vi "Fixated.vi"(10 "Input":variant, 11 "Data":T1) -> (2 "Fixated":bool, 3 "Adjustment":dbl[](array[numeric]))   [LabVIEW 2010]
uses:
  Core SubVIs/Controls/TYPE - Analog Data.ctl
  <vilib>/imath/engines/lvmath2/RunTimeEngine/ErrorHandling/NIMS_Finalize Error.vi
  <vilib>/imath/engines/lvmath2/RunTimeEngine/NodeEndStatement/NIMS_NodeEndStatement_Output.vi
  <instcachedir>/0/NIMS_NodeEndStatement_Output_53EC0D466D134D7ABD903AC30B43404B.lvgen/NIMS_NodeEndStatement_Output_53EC0D466D134D7ABD903AC30B43404B_009.vi
  <vilib>/imath/engines/lvmath2/RunTimeEngine/ArithmeticOperatorToken/NIMS_ArithmeticOperator_plus.vi
  <instcachedir>/0/NIMS_ArithmeticOperator_plus_5FA379184E244F92A148919B9FCD7B31.lvgen/NIMS_ArithmeticOperator_plus_5FA379184E244F92A148919B9FCD7B31_004.vi
  <vilib>/imath/engines/lvmath2/RunTimeEngine/BuiltInFunctions/mean/NIMS_CS=mean(CV,I32).vi
  <vilib>/imathl/engines/lvmath/Functions/Error Handling/Create Error.vi
  Core SubVIs/Core SubVIs.lvlib
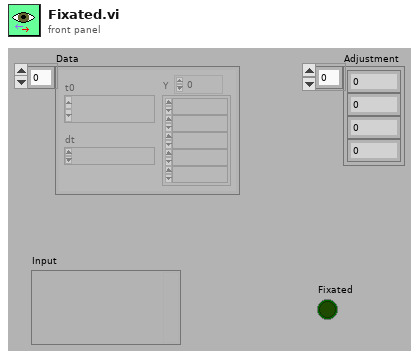
[diagram p1: front panel]
types:
  T1 = typedef "Core SubVIs.lvlib/TYPE - Analog Data.ctl" = waveform(dbl)[]
  T2 = cluster{"Trial Type":i32, "Joystick Threshold":dbl, "Fixation Radius":dbl}
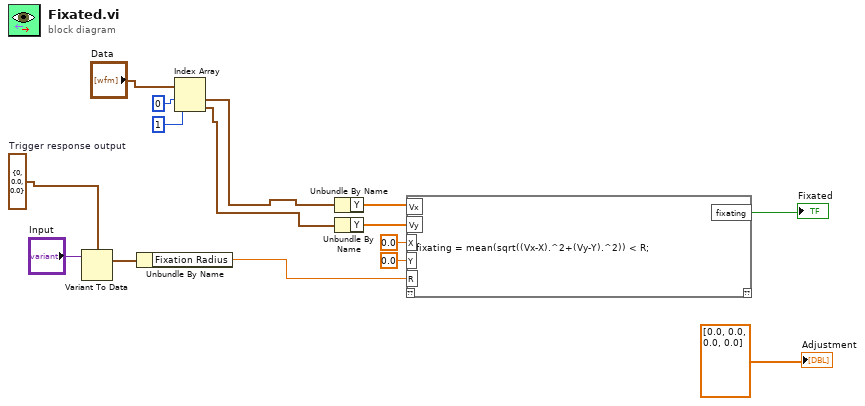
[diagram p0: block diagram]
diagram:
  w1 = T2 {"Trial Type"=0, "Joystick Threshold"=0.0, "Fixation Radius"=0.0}  # Trigger response output
  n1 = Variant To Data(Variant="Input", type=w1) -> (data=w3:T2)  [unwired: 1 in, 1 out]
  n2 = Unbundle By Name(w3) -> ("Fixation Radius"=w2:dbl)
  n3 = Index Array(array="Data", index #1=0 ("index"), index #2=1 ("index")) -> (element #1=w7:waveform(dbl), element #2=w6:waveform(dbl))
  n4 = Unbundle By Name(w7) -> ("Y"=w12:dbl[])
  n5 = Unbundle By Name(w6) -> ("Y"=w11:dbl[])
  n6 = mathscript code="fixating = mean(sqrt((Vx-X).^2+(Vy-Y).^2)) < R;"("Vx"=w12, "Vy"=w11, "X"=0.0, "Y"=0.0, "R"=w2) -> ("fixating"=→"Fixated":bool)  [unwired: 1 in, 1 out]
  "Adjustment" <- dbl[] [0.0, 0.0, 0.0, 0.0] ("Adjustment")
